vi "SMO.jsonRPC.SendAsynchronousCommand.vi"(6 "timeout (50ms)":i32=50, 7 "Notification (F)":bool, 8 "error in (no error)":errorcluster, 9 "Parameters":variant, 10 "Method":string, 11 "SMO.jsonRPC in":refnum<class "SMO.jsonRPC.lvclass">) -> (0 "error out":errorcluster, 1 "id":i32, 2 "Response":refnum<class "Response.lvclass">, 3 "SMO.jsonRPC out":refnum<class "SMO.jsonRPC.lvclass">)   [LabVIEW 2013, in "SMO.jsonRPC.lvclass"]
uses:
  SMO.jsonRPC.lvclass
  <vilib>/JKI/JKI JSON RPC Specification/Response/Response.lvclass
  Typedefs/Request--Cluster.ctl
  <vilib>/JKI/JKI JSON RPC Specification/Request/Request.lvclass
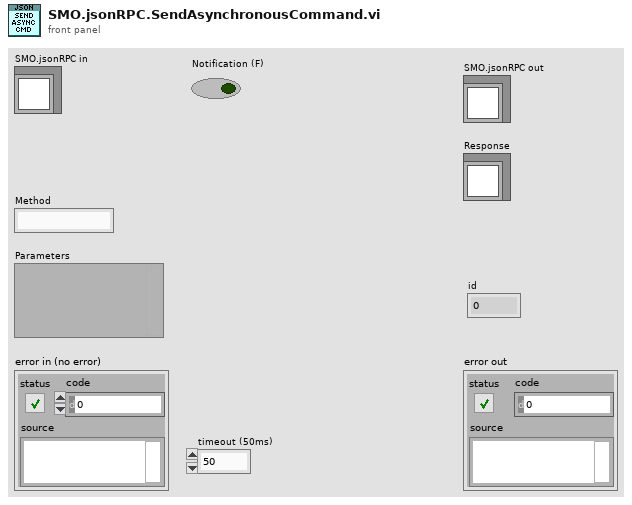
[diagram p1: front panel]
types:
  T1 = typedef "SMO.jsonRPC.lvclass/Request--Cluster.ctl" = cluster{"Request":refnum<class "Request.lvclass">, "reply queue":refnum<queue>, "Async?":bool}
  T2 = typedef "SMO.jsonRPC.lvclass/PrivateEvents--Cluster.ctl" = cluster{"Incoming Request":refnum<user-event>}
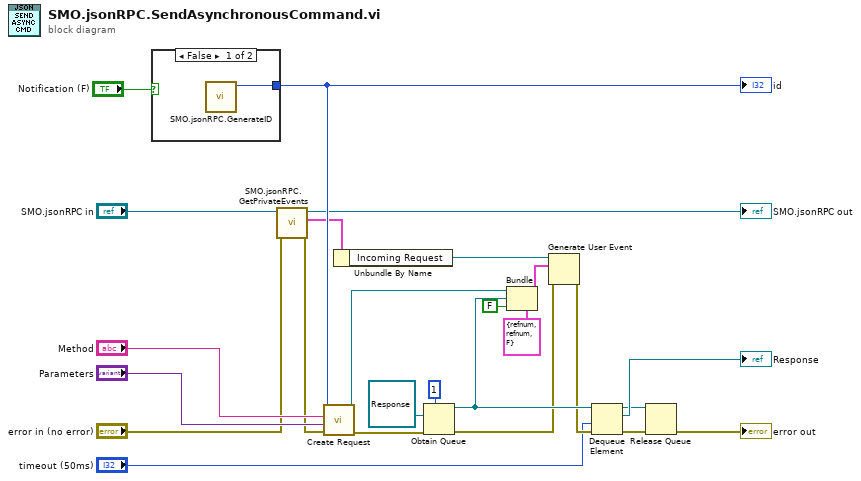
[diagram p0: block diagram]
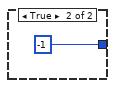
[diagram p2: hidden frame]
diagram:
  n1 = case shown="False" "Notification (F)" {
    tunnel: [w26 -1 ("id")] -> w25
    frame False {
      n2 = call "SMO.jsonRPC.GenerateID.vi"() -> ("id"=w26:i32)  [unwired: 11 in]
    }
    frame True {
    }
  }
  "id" <- w25
  n3 = call "SMO.jsonRPC.GetPrivateEvents.vi"("error in (no error)"="error in (no error)", "SMO.jsonRPC"="SMO.jsonRPC in") -> ("error out"=w19:errorcluster, "Private Events"=w4:T2, "SMO.jsonRPC out"=→"SMO.jsonRPC out":refnum<class "SMO.jsonRPC.lvclass">)  [unwired: 7 in]
  n4 = call <vilib>:"Create Request.vi"("error in (no error)"=w19, "Parameters"="Parameters", "Method"="Method", "id (-1: notification)"=w25) -> ("error out"=w17:errorcluster, "Request"=w16:refnum<class "Request.lvclass">)  [unwired: 5 in, 1 out]
  n5 = Unbundle By Name(w4) -> ("Incoming Request"=w3:refnum<user-event>)
  n6 = Obtain Queue(max queue size (-1, unlimited)=1, element data type=refnum<class "Response.lvclass"> refnum ("Response"), error in (no error)=w17) -> (queue out=w13:refnum<queue>, error out=w7:errorcluster)  [unwired: 2 in, 1 out]
  n7 = Bundle(cluster=T1 {"Request"=refnum, "reply queue"=refnum, "Async?"=FALSE} ("event data"), "Request"=w16, "reply queue"=w13, "Async?"=FALSE) -> (w6:T1)
  n8 = Generate User Event(user event=w3, event data cluster=w6, error in=w7) -> (error out=w11:errorcluster)  [unwired: 1 in, 1 out]
  n9 = Dequeue Element(queue=w13, timeout in ms (-1)="timeout (50ms)", error in (no error)=w11) -> (queue out=w9:refnum<queue>, element=→"Response":refnum<class "Response.lvclass">, error out=w10:errorcluster)  [unwired: 1 out]
  n10 = Release Queue(queue=w9, error in (no error)=w10) -> (error out=→"error out":errorcluster)  [unwired: 1 in, 2 out]
